vi "Read SetGratingType.vi"(8 "error in (no error)":errorcluster, 11 "MonoPubSubData in":refnum<class "MonoPubSubData.lvclass">) -> (0 "error out":errorcluster, 2 "SetGratingType":refnum<user-event>, 3 "MonoPubSubData out":refnum<class "MonoPubSubData.lvclass">)   [LabVIEW 2016, in "MonoPubSubData.lvclass"]
uses:
  MonoPubSubData.lvclass
  Typedefs/GratingType.ctl
  MonoPubSubData.lvclass/MonoPubSubData.ctl
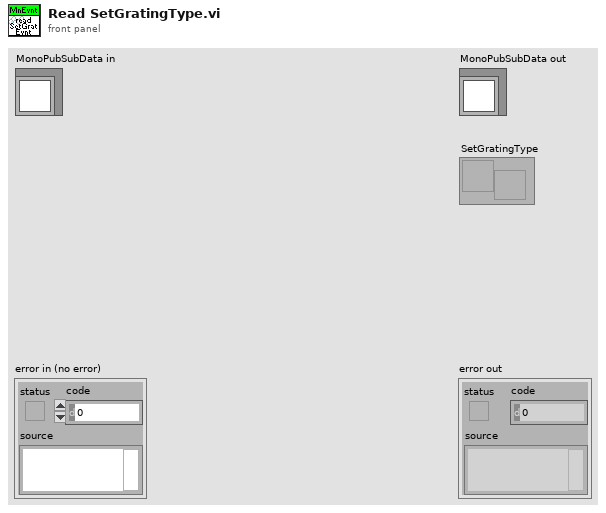
[diagram p1: front panel]
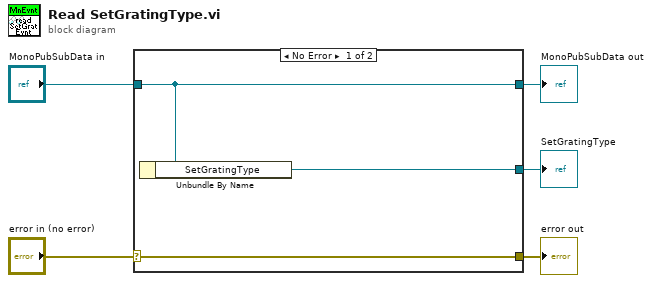
[diagram p0: block diagram]
diagram:
  n1 = case shown="No Error" "error in (no error)" {
    selector: "error in (no error)" -> [w8 w9]
    tunnel: [w8 w9] -> w4
    tunnel: [w7 w10] -> w2
    tunnel: "MonoPubSubData in" -> [w7 w10]
    tunnel: [w6 _] -> w1
    frame No Error {
      n2 = Unbundle By Name(w7) -> ("SetGratingType"=w6:refnum<user-event>)
    }
    frame Error {
    }
  }
  "error out" <- w4
  "MonoPubSubData out" <- w2
  "SetGratingType" <- w1
